vi "run.vi"(8 "error in (no error)":errorcluster, 11 "ImagingModeDL090130Frame in":refnum<class "ImagingModeDL090130Frame.lvclass">=refnum) -> (0 "error out":errorcluster, 3 "ImagingModeDL090130Frame out":refnum<class "ImagingModeDL090130Frame.lvclass">)   [LabVIEW 2010, in "ImagingModeDL090130Frame.lvclass"]
uses:
  ImagingModeDL090130Frame.lvclass
  internal_trigger_enum.ctl
  main/labview_source/controls/undock_button.ctl
  translation_mode_enum.ctl
  common/xcontrols/XSettings/XSettings/XSettings.xctl
  common/classes/GenericComponent/GenericComponent/GenericComponent.lvclass
  common/xcontrols/XIntensityCompensation/XIntensityCompensation/XIntensityCompensation.xctl
  speed_constant_enum.ctl
  control_refs.ctl
  state_enum.ctl
  common/classes/GenericToplevelComponent/GenericToplevelComponent/trigger_type_enum.ctl
  GenericImagingMode/GenericImagingMode/GenericImagingMode.lvclass
  ImagingModeDL090130Frame.lvclass/ImagingModeDL090130Frame.ctl
  Trajectory/GenericTrajectory/GenericTrajectory/GenericTrajectory.lvclass
  common/classes/ErrorController/ErrorController/class_data.vi
  common/classes/ErrorController/ErrorController/ErrorController.lvclass
panel:
  out "enforce settings?":bool
  in  "button:undock":T1
  in  "Tab Control":enum32{"User", "Debug", "About"}(tab)
  in  "amplitude\n (y galvo, V)":dbl(slide)=1.0 min=0.0 max=4.0 step=0.01 scale=0.0..4.0
  in  "center\n (y galvo, V)":dbl(slide) min=-2.0 max=2.0 step=0.01 scale=-2.0..2.0
  in  "amplitude\n (x galvo, V)":dbl(slide)=1.0 min=0.0 max=4.0 step=0.01 scale=0.0..4.0
  in  "center\n (x galvo, V)":dbl(slide)=1.1102230246251565e-16 min=-2.0 max=2.0 step=0.01 scale=-2.0..2.0
  in  "XIntensityCompensation":cluster{"A":dbl, "lambda":dbl[unit], "C":dbl}(xcontrol)
  in  "translation mode":T2
  in  "return to origin?":bool=TRUE
  in  "step":dbl[unit] min=0.0 max=0.01 step=1e-07
  in  "no. of averagings":i32=1 caption="repetitions/\naveraging" min=1 max=100000000
  in  "movie duration":dbl[unit]=10.24 min=0.0 max=3600.0
  in  "no. of frames":i32=20 caption="frames" min=1 max=100000
  in  "defineButton":bool
  in  "frame rate":dbl[unit]=1.953125 min=0.0 max=100.0
  in  "pixel dwell time":dbl[unit]=7.8125e-06 min=0.0 max=0.001
  in  "line scan time":dbl[unit]=0.002 min=0.0 max=1.0
  in  "y aspect":dbl=1.0 caption=":" min=0.0
  in  "x aspect":dbl=1.0 caption="aspect ratio (x:y)" min=0.0 step=1.0
  in  "y lines":i32=256 min=0 max=1000
  out "offset":dbl[unit]
  in  "x pixels":i32=256 min=0 max=1000 step=1
  out "frame no.":i32=12 caption="frame"
  out "repetition no.":i32=1 caption="repetition"
  in  "settings":refnum<class "GenericComponent.lvclass">(xcontrol)
  in  "keep constant":T3
  out "Vmax(ygalvo)":dbl
  out "Vmin(ygalvo)":dbl
  out "Vmax(xgalvo)":dbl
  out "Vmin(xgalvo)":dbl
  in  "xy galvo view?":bool
  out "event handling loop counter":i32=10
  out "statemachine loop counter":i32=75
  out "event error":errorcluster
  out "action handler error":errorcluster
  out "finished?":bool
  out "last trigger":T4
  out "internal triggers":T4[](array[typedef])
  # "stack settings"
  # "y galvo:"
  # "frame settings"
  # "TAG lens:"
  # "x galvo:"
  # "in fact 2x"
  # "current values"
  # "if no extra lines\nframe rate x2"
  # "ImagingModeDL090130Frame"
  # "Implemented by: \nDominik Langer, University of Zurich"
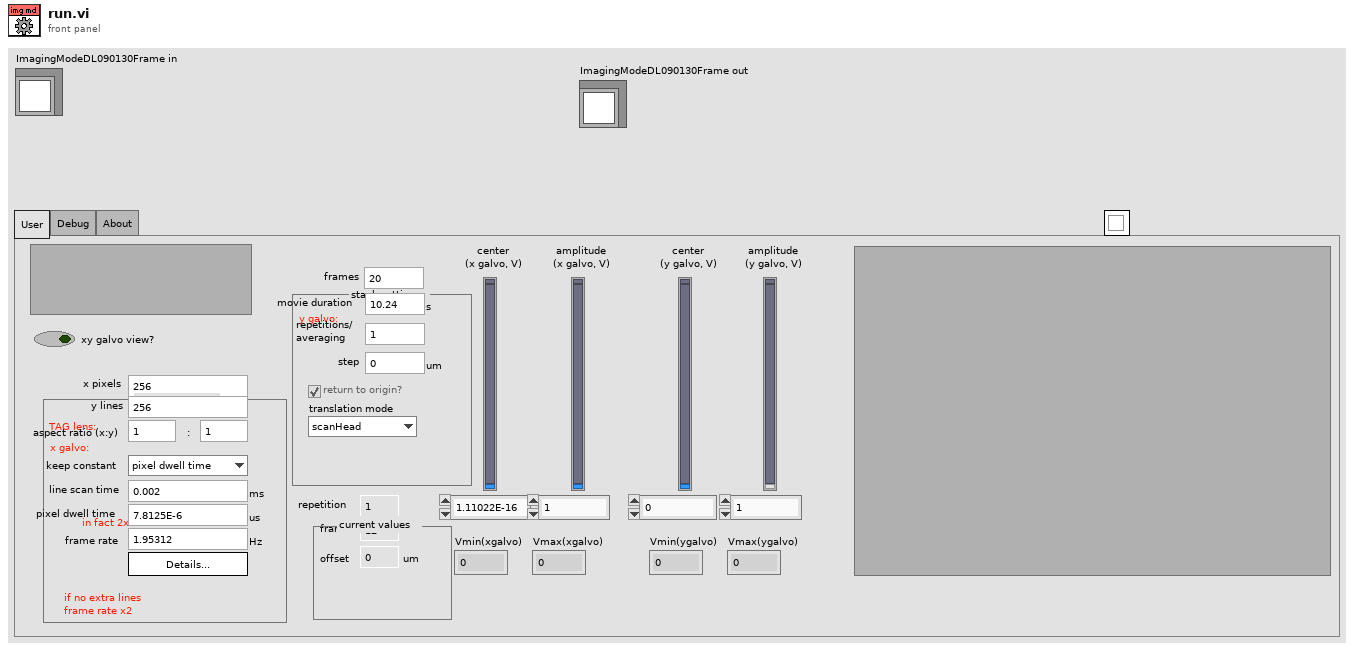
[diagram p1: front panel]
types:
  T1 = typedef "undock_button.ctl" = bool
  T2 = typedef "ImagingModeDL090130Frame.lvclass/translation_mode_enum.ctl" = enum16{"scanHead", "stage"}
  T3 = typedef "ImagingModeDL090130Frame.lvclass/speed_constant_enum.ctl" = enum16{"pixel dwell time", "line scan time", "frame rate"}
  T4 = typedef "ImagingModeDL090130Frame.lvclass/internal_trigger_enum.ctl" = enum16{"NULL", "initialise", "terminate", "start", "stop", "proceed", "update", "translate", "start scanning"}
  T5 = typedef "ImagingModeDL090130Frame.lvclass/control_refs.ctl" = cluster{"resolution controls":cluster{"x pixels":refnum<vi>, "y pixels":refnum<vi>, "ratio x factor":refnum<vi>, "ratio y factor":refnum<vi>, "center(xgalvo,V)":refnum<vi>, "center(ygalvo,V)":refnum<vi>, "amplitude(ygalvo,V)":refnum<vi>, "amplitude(xgalvo,V)":refnum<vi>, "xy galvo view?":refnum<vi>}, "speed controls":cluster{"pixel dwell time":refnum<vi>, "line scan time":refnum<vi>, "frame rate":refnum<vi>, "keep constant":refnum<vi>}, "number of frames controls":cluster{"# of frames":refnum<vi>, "duration":refnum<vi>, "# of repetitions":refnum<vi>}, "current value indicators":cluster{"frame #":refnum<vi>, "repetition #":refnum<vi>, "offset":refnum<vi>}, "step controls":cluster{"step size":refnum<vi>, "return to origin?":refnum<vi>, "translation mode":refnum<vi>, "XIntensityCompensation":refnum<vi>}, "defineButton":refnum<vi>, "settings enforced?":refnum<vi>, "settings":refnum<vi>}
  T6 = typedef "ImagingModeDL090130Frame.lvclass/state_enum.ctl" = enum16{"idle", "sweep (scanning)", "sweep (translating)"}
  T7 = typedef "trigger_type_enum.ctl" = enum8{"external", "internal", "common"}
  T8 = typedef "main_trigger_enum.ctl" = enum16{"NULL", "initialise", "terminate", "start", "stop", "change objective", "change experimentController", "change imagingMode", "save notebook", "started saving", "finished saving", "expCtr ready", "expCtr missing", "imgMd ready", "imgMd missing", "scanHd ready", "scanHd missing", "DAQ ready", "DAQ missing", "imgAsm ready", "imgAsm missing", "dataColl ready", "dataColl missing", "display ready", "display missing", "analysr ready", "analysr missing", "instrmnt ready", "instrmnt missing", "stimltr ready", "stimltr missing", "stage ready", "stage missing"}
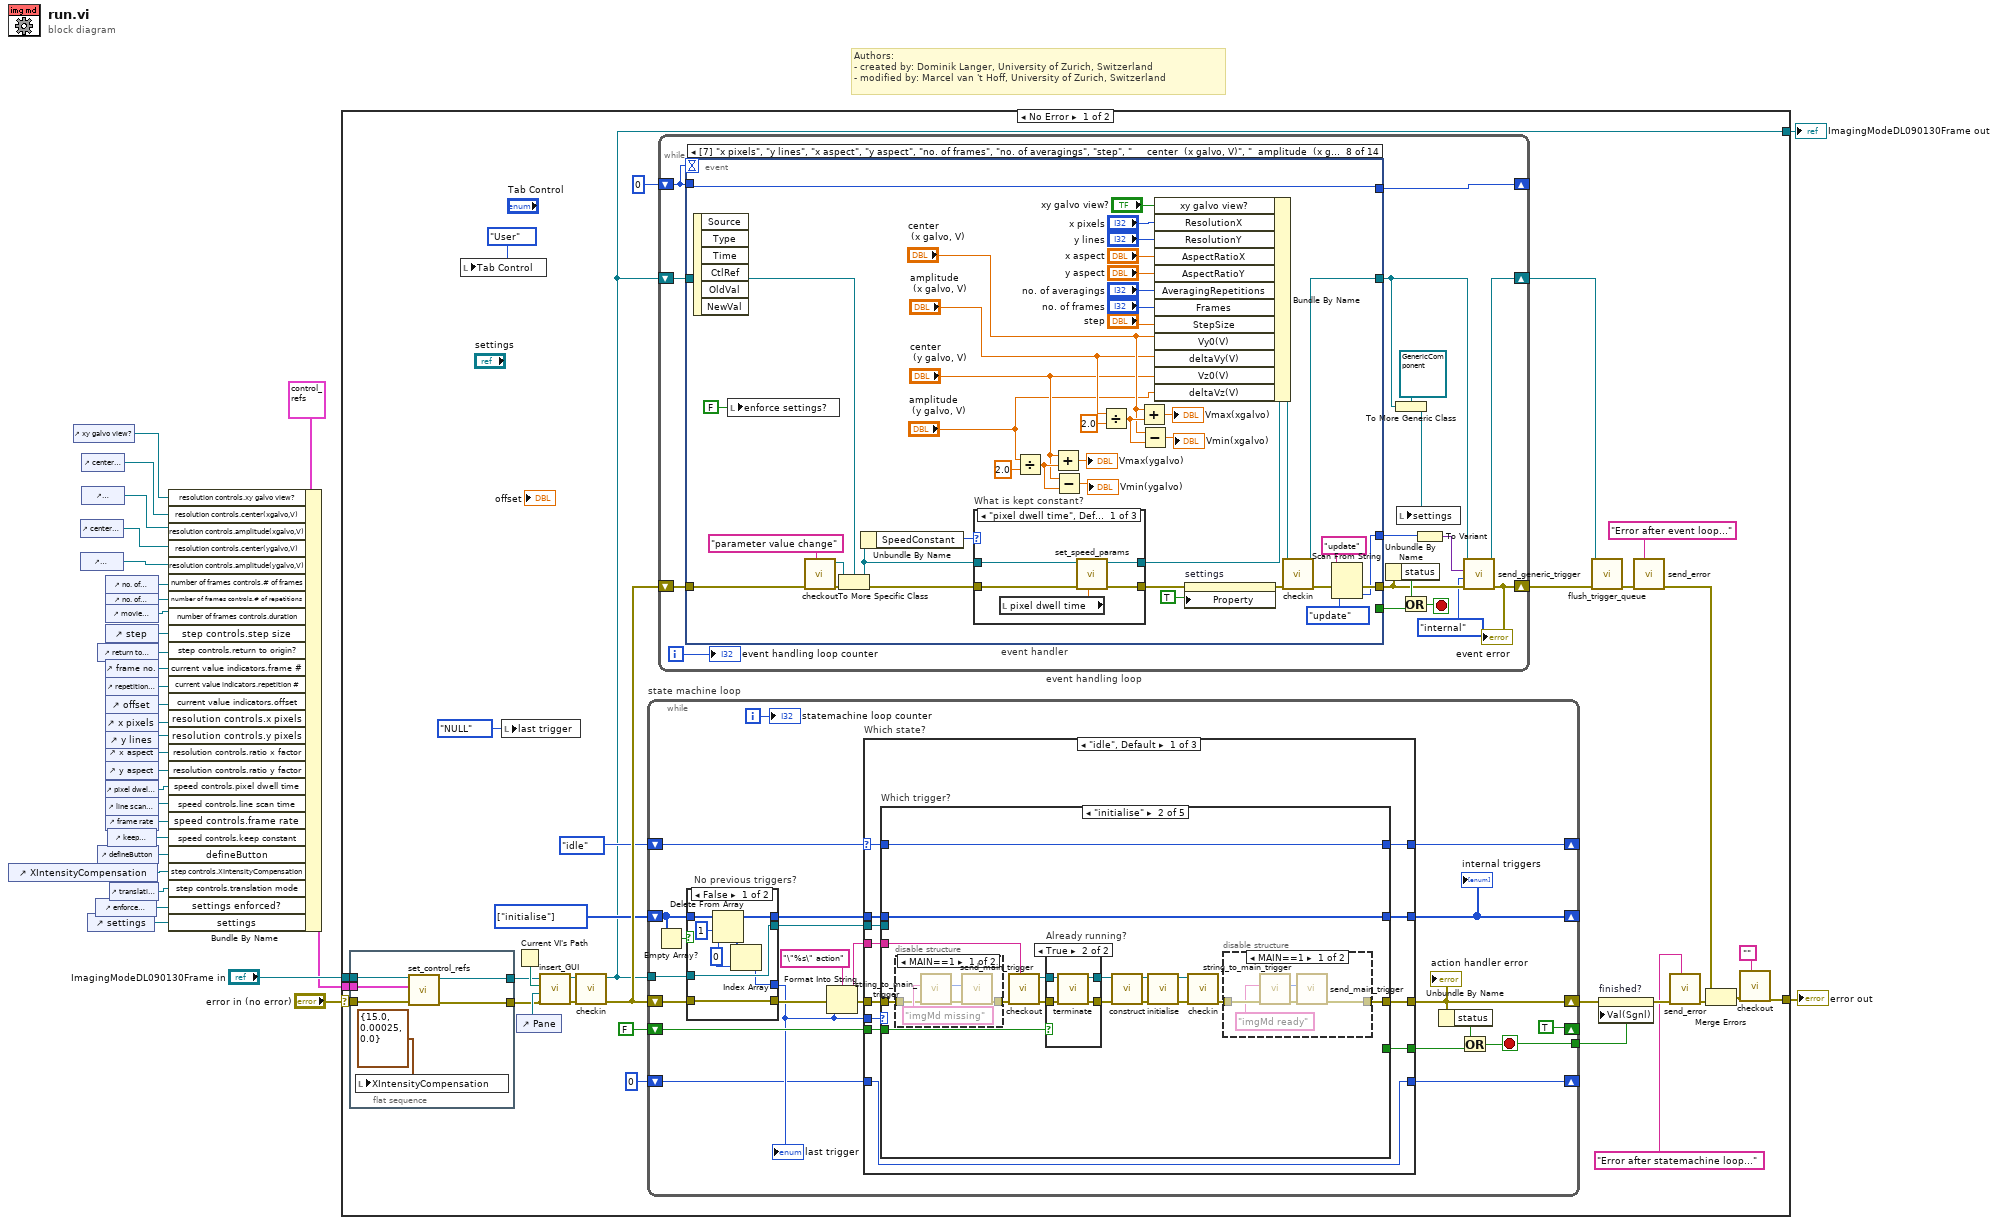
[diagram p0: block diagram]
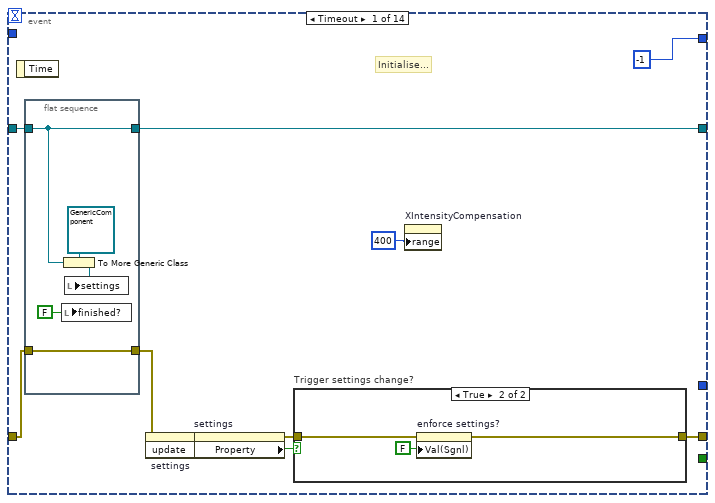
[diagram p2: hidden frame]
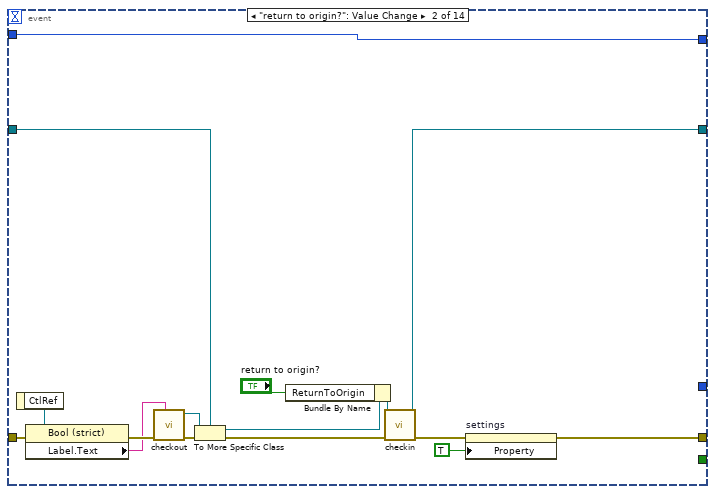
[diagram p4: hidden frame]
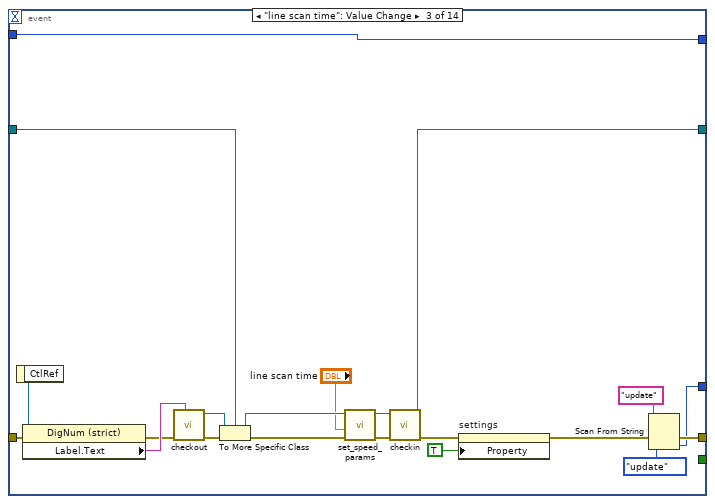
[diagram p5: hidden frame]
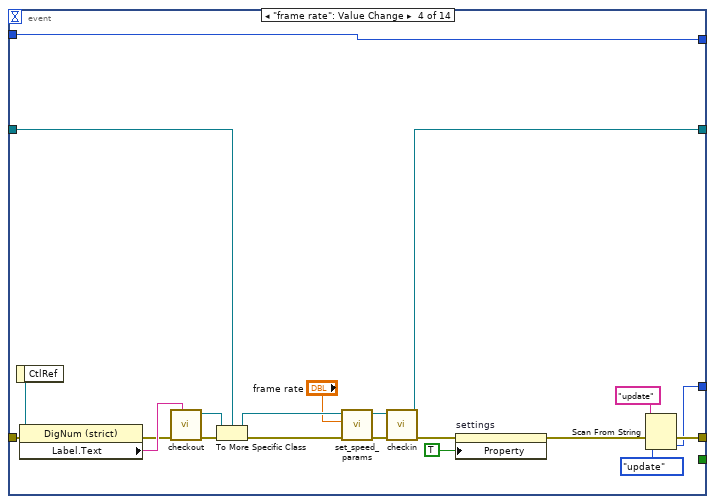
[diagram p6: hidden frame]
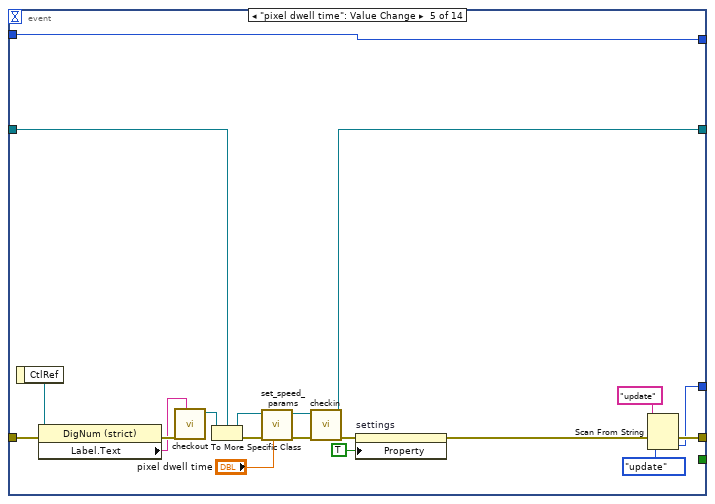
[diagram p7: hidden frame]
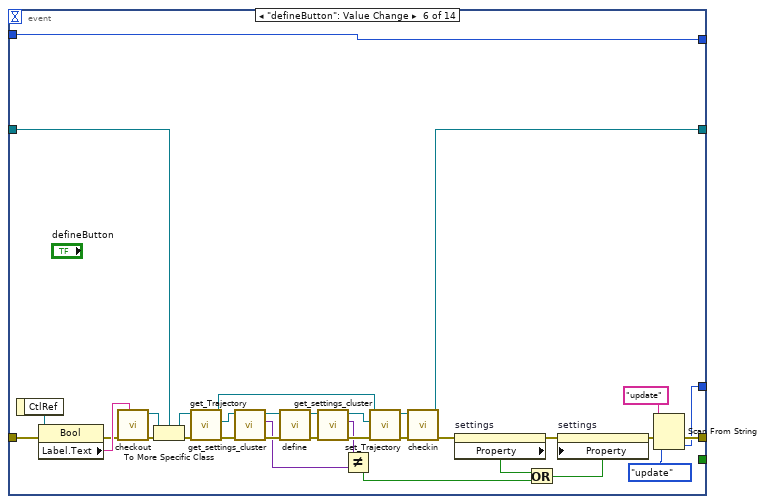
[diagram p8: hidden frame]
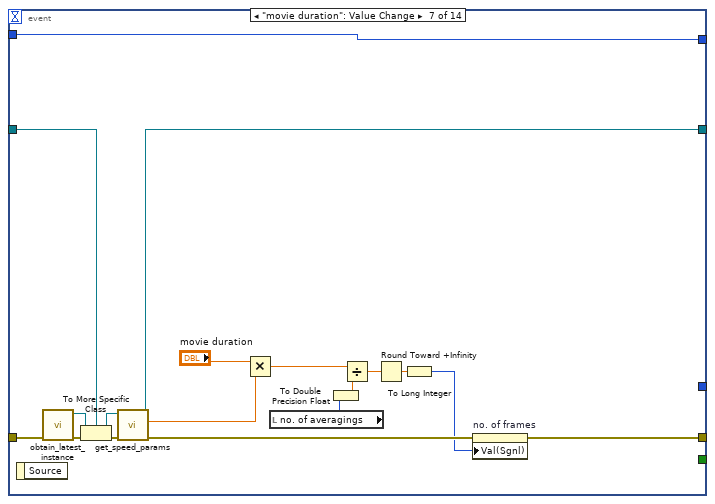
[diagram p9: hidden frame]
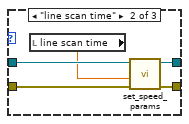
[diagram p10: hidden frame]
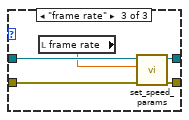
[diagram p11: hidden frame]
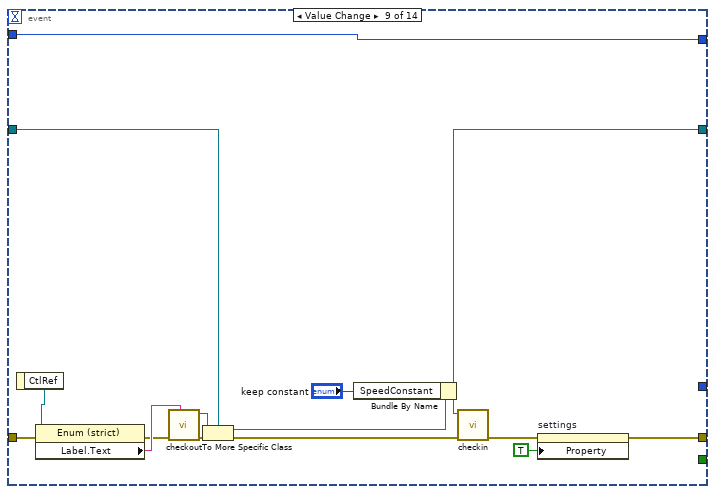
[diagram p12: hidden frame]
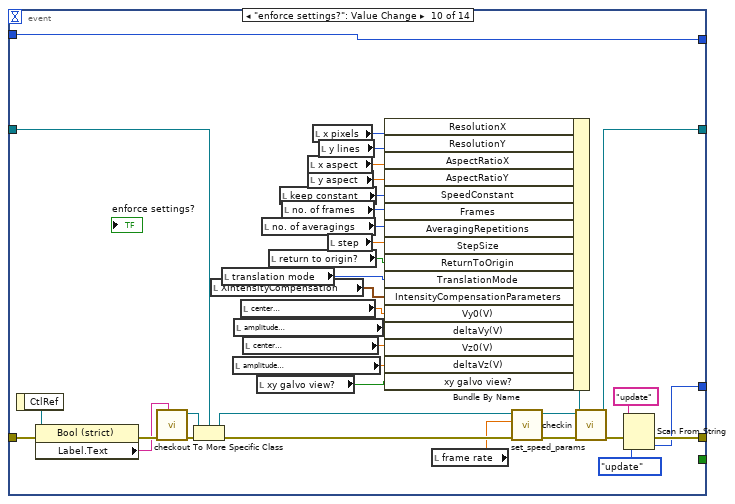
[diagram p13: hidden frame]
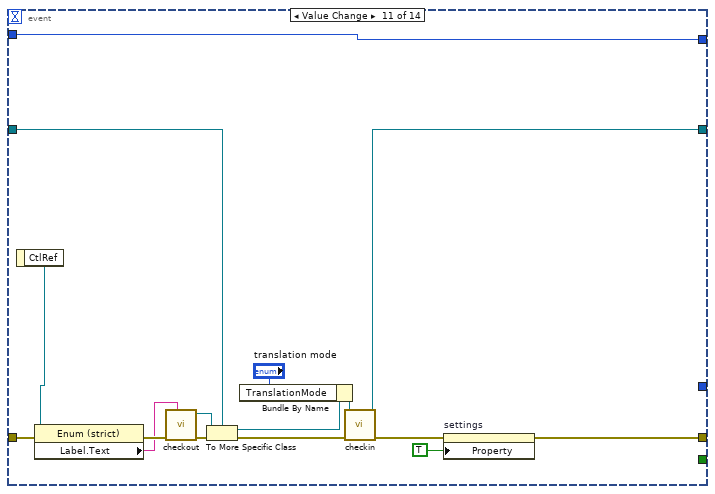
[diagram p14: hidden frame]
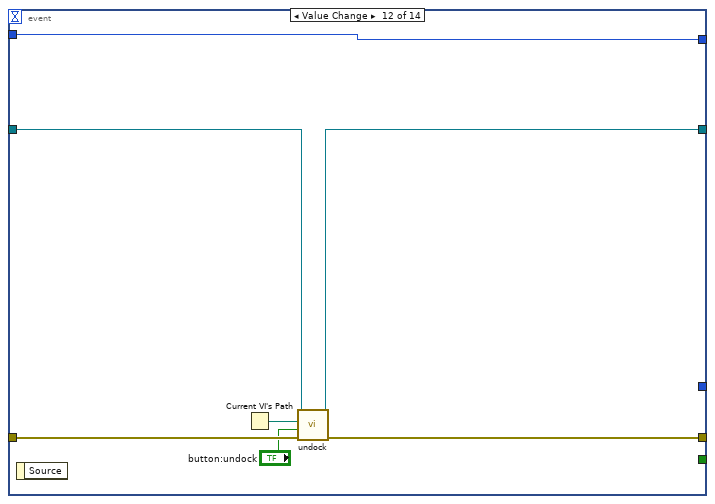
[diagram p15: hidden frame]
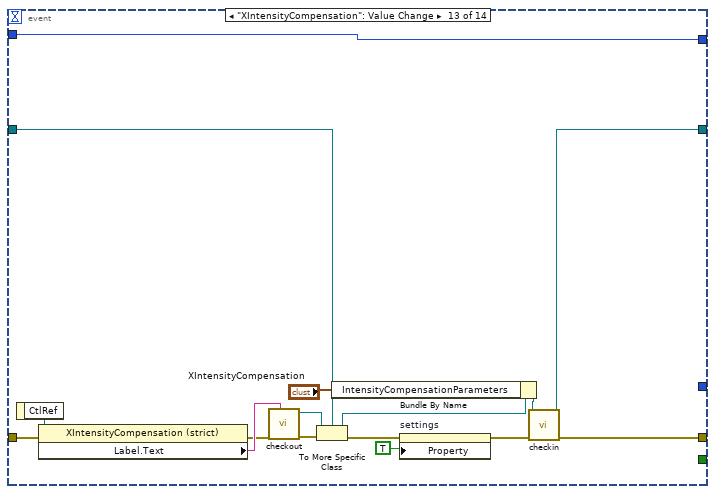
[diagram p16: hidden frame]
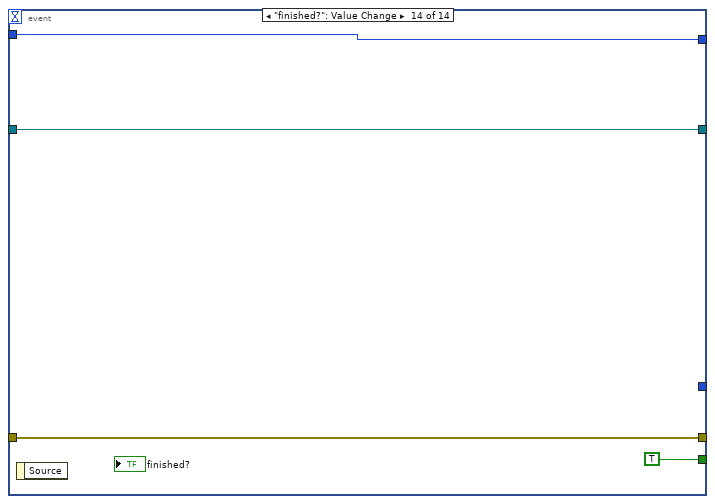
[diagram p17: hidden frame]
diagram:
  # "Authors: \n- created by: Dominik Langer, University of Zurich, Switzerland\n- modified by: Marcel van 't Hoff, University of Zurich, Switzerland"
  n1 = control-ref of="XIntensityCompensation"() -> (w10:refnum<vi>)
  n2 = control-ref of="xy galvo view?"() -> (w1:refnum<vi>)
  n3 = control-ref of="center\n (y galvo, V)"() -> (w4:refnum<vi>)
  n4 = control-ref of="amplitude\n (y galvo, V)"() -> (w3:refnum<vi>)
  n5 = control-ref of="center\n (x galvo, V)"() -> (w2:refnum<vi>)
  n6 = control-ref of="amplitude\n (x galvo, V)"() -> (w5:refnum<vi>)
  n7 = control-ref of="settings"() -> (w6:refnum<vi>)
  n8 = control-ref of="enforce settings?"() -> (w8:refnum<vi>)
  n9 = control-ref of="return to origin?"() -> (w11:refnum<vi>)
  n10 = control-ref of="defineButton"() -> (w20:refnum<vi>)
  n11 = control-ref of="no. of frames"() -> (w16:refnum<vi>)
  n12 = control-ref of="no. of averagings"() -> (w14:refnum<vi>)
  n13 = control-ref of="movie duration"() -> (w15:refnum<vi>)
  n14 = control-ref of="step"() -> (w13:refnum<vi>)
  n15 = control-ref of="frame no."() -> (w27:refnum<vi>)
  n16 = control-ref of="repetition no."() -> (w28:refnum<vi>)
  n17 = control-ref of="offset"() -> (w30:refnum<vi>)
  n18 = control-ref of="x pixels"() -> (w29:refnum<vi>)
  n19 = control-ref of="y lines"() -> (w23:refnum<vi>)
  n20 = control-ref of="x aspect"() -> (w22:refnum<vi>)
  n21 = control-ref of="y aspect"() -> (w21:refnum<vi>)
  n22 = control-ref of="pixel dwell time"() -> (w17:refnum<vi>)
  n23 = control-ref of="line scan time"() -> (w18:refnum<vi>)
  n24 = control-ref of="frame rate"() -> (w19:refnum<vi>)
  n25 = control-ref of="keep constant"() -> (w7:refnum<vi>)
  n26 = control-ref of="translation mode"() -> (w12:refnum<vi>)
  n27 = Bundle By Name(cluster=T5 {"resolution controls"={"x pixels"=refnum, "y pixels"=refnum, "ratio x factor"=refnum, "ratio y factor"=refnum, "center(xgalvo,V)"=refnum, "center(ygalvo,V)"=refnum, "amplitude(ygalvo,V)"=refnum, "amplitude(xgalvo,V)"=refnum, "xy galvo view?"=refnum}, "speed controls"={"pixel dwell time"=refnum, "line scan time"=refnum, "frame rate"=refnum, "keep constant"=refnum}, "number of frames controls"={"# of frames"=refnum, "duration"=refnum, "# of repetitions"=refnum}, "current value indicators"={"frame #"=refnum, "repetition #"=refnum, "offset"=refnum}, "step controls"={"step size"=refnum, "return to origin?"=refnum, "translation mode"=refnum, "XIntensityCompensation"=refnum}, "defineButton"=refnum, "settings enforced?"=refnum, "settings"=refnum} ("control refs"), "resolution controls.xy galvo view?"=w1, "resolution controls.center(xgalvo,V)"=w2, "resolution controls.amplitude(xgalvo,V)"=w5, "resolution controls.center(ygalvo,V)"=w4, "resolution controls.amplitude(ygalvo,V)"=w3, "number of frames controls.# of frames"=w16, "number of frames controls.# of repetitions"=w14, "number of frames controls.duration"=w15, "step controls.step size"=w13, "step controls.return to origin?"=w11, "current value indicators.frame #"=w27, "current value indicators.repetition #"=w28, "current value indicators.offset"=w30, "resolution controls.x pixels"=w29, "resolution controls.y pixels"=w23, "resolution controls.ratio x factor"=w22, "resolution controls.ratio y factor"=w21, "speed controls.pixel dwell time"=w17, "speed controls.line scan time"=w18, "speed controls.frame rate"=w19, "speed controls.keep constant"=w7, "defineButton"=w20, "step controls.XIntensityCompensation"=w10, "step controls.translation mode"=w12, "settings enforced?"=w8, "settings"=w6) -> (w24:T5)
  n28 = case shown="No Error" "error in (no error)" {
    selector: "error in (no error)" -> [w48 w659]
    tunnel: [w51 w659] -> w32
    tunnel: [w35 w658] -> w31
    tunnel: "ImagingModeDL090130Frame in" -> [w44 w658]
    tunnel: w24 -> [w45 _]
    frame No Error {
      w39 = T4[] [enum."initialise"] items=["NULL", "initialise", "terminate", "start", "stop", "proceed", "update", "translate", "start scanning"]
      n29 = flat-sequence {
        tunnel: w48 -> [w69]
        tunnel: [w68] -> w47
        tunnel: [w67] -> w46
        tunnel: w45 -> [w66]
        tunnel: w44 -> [w65]
        frame #0 {
          n30 = local write "XIntensityCompensation"(cluster{"A":dbl, "lambda":dbl[unit], "C":dbl} {"A"=15.0, "lambda"=0.00025, "C"=0.0} ("XIntensityCompensation")) -> ()
          n31 = call "set_control_refs.vi"("error in (no error)"=w69, "control refs"=w66, "ImagingModeDL090130Frame in"=w65) -> ("error out"=w67:errorcluster, "ImagingModeDL090130Frame out"=w68:refnum<class "ImagingModeDL090130Frame.lvclass">)  [unwired: 7 in]
        }
      }
      n32 = local write "Tab Control"(enum32{"User", "Debug", "About"}."User" ("Tab Control")) -> ()
      n33 = local write "last trigger"(internal_trigger_enum."NULL" ("last trigger")) -> ()
      n34 = Current VI's Path() -> (path=w59:path)
      n35 = control-ref of="Pane"() -> (w57:refnum<vi>)
      n36 = call-dynamic "insert_GUI.vi"("error in (no error)"=w46, "Pane"=w57, "VI path"=w59, "GenericComponent in"=w47) -> ("error out"=w34:errorcluster, "GenericComponent out"=w43:refnum<class "ImagingModeDL090130Frame.lvclass">)  [unwired: 6 in]
      n37 = call-dynamic "checkin.vi"("error in (no error)"=w34, "GenericScanMode in"=w43) -> ("error out"=w60:errorcluster, "GenericScanMode out"=w35:refnum<class "ImagingModeDL090130Frame.lvclass">)  [unwired: 8 in]
      n38 = while "state machine loop" {
        shift-right: [TRUE] -> _
        shift-left: FALSE -> [w396]
        tunnel: w35 -> [w407]
        tunnel: [w405] -> w42
        shift-right: [w402] -> w61
        shift-left: w60 -> [w406]
        shift-right: [w392] -> _
        shift-left: w39 -> [w394]
        shift-right: [w390] -> _
        shift-left: state_enum."idle" ("state") -> [w391]
        shift-right: [w386] -> _
        shift-left: u32 0 ("millisecond timer value") -> [w387]
        i -> [w388]
        stop <- w405 stop-if-true
        n39 = Empty Array?(array=w394) -> (empty?=w395:bool)
        n40 = case "No previous triggers?" shown="False" w395 {
          tunnel: w407 -> [w649 w657]
          tunnel: w406 -> [w651 w656]
          tunnel: [w649 w655] -> w404
          tunnel: [w644 w654] -> w389
          tunnel: [w651 w653] -> w400
          tunnel: w394 -> [w650 w652]
          tunnel: [w647 w652] -> w393
          frame False {
            w645 = 0 ("index")
            n41 = Delete From Array(array=w650, length=1, index=w645) -> (deleted portion=w646:T4[], array with subset deleted=w647:T4[])
            n42 = Index Array(array=w646, index=w645) -> (element=w644:T4)
          }
          frame True {
            n43 = call-dynamic "fetch_and_translate_trigger.vi"("error in (no error)"=w656, "ImagingModeDL090130Frame in"=w657) -> ("error out"=w653:errorcluster, "internal trigger"=w654:T4, "ImagingModeDL090130Frame out"=w655:refnum<class "ImagingModeDL090130Frame.lvclass">)  [unwired: 6 in, 1 out]
          }
        }
        "last trigger" <- w389
        n44 = Format Into String(format string="\"%s\" action", error in=w400, w389) -> (resulting string=w398:string, error out=w399:errorcluster)  [unwired: 1 in]
        n45 = case "Which state?" shown="\"idle\", Default" w391 {
          selector: w391 -> [w411 w505 w616]
          tunnel: w404 -> [w420 w508 w609]
          tunnel: [w419 _ _] -> w403
          tunnel: [w418 w510 w611] -> w402
          tunnel: w399 -> [w417 w511 w613]
          tunnel: w398 -> [w416 w507 w608]
          tunnel: w396 -> [w415 _ _]
          tunnel: w393 -> [w414 w509 w614]
          tunnel: w389 -> [w413 w503 w612]
          tunnel: [w412 w506 w610] -> w392
          tunnel: [w410 w504 w615] -> w390
          tunnel: w387 -> [w409 w502 w607]
          tunnel: [w409 w501 w607] -> w386
          frame "idle", Default {
            n46 = case "Which trigger?" shown="\"initialise\"" w413 {
              tunnel: w417 -> [w423 w425 w461 w482 w492]
              tunnel: w420 -> [_ _ _ w479 w490]
              tunnel: [w423 w427 w459 w481 w491] -> w418
              tunnel: [_ _ TRUE _ _] -> w419
              tunnel: w414 -> [w422 w439 w467 w478 w500]
              tunnel: [w422 w439 w467 w477 w500] -> w412
              tunnel: w416 -> [_ w436 w462 w480 w493]
              tunnel: w415 -> [_ w429 _ _ _]
              tunnel: [w421 w426 w458 state_enum."sweep (scanning)" ("state") w489] -> w410
              tunnel: w411 -> [w421 w426 w458 _ w489]
              frame "NULL", Default {
              }
              frame "initialise" {
                n47 = disable-structure shown="MAIN==1" {
                  disable-tunnel: w425 -> [w440 w445]
                  disable-tunnel: [w444 w445] -> w424
                  frame condition #0 {
                    n48 = call "string_to_main_trigger.vi"("error in (no error)"=w440, "trigger string"="imgMd missing") -> ("error out"=w443:errorcluster, "main trigger"=w442:T8)  [unwired: 8 in]
                    n49 = call "send_main_trigger.vi"("error in (no error)"=w443, "trigger"=w442) -> ("error out"=w444:errorcluster)  [unwired: 9 in]
                  }
                  frame condition #1 (active) {
                  }
                }
                n50 = call "checkout.vi"("locked by?"=w436, "error in (no error)"=w424) -> ("error out"=w433:errorcluster, "GenericScanMode out"=w432:refnum<class "GenericImagingMode.lvclass">)  [unwired: 8 in]
                n51 = case "Already running?" shown="True" w429 {
                  tunnel: w433 -> [w453 w457]
                  tunnel: w432 -> [w452 w456]
                  tunnel: [w452 w455] -> w431
                  tunnel: [w453 w454] -> w430
                  frame False {
                  }
                  frame True {
                    n52 = call-dynamic "terminate.vi"("error in (no error)"=w457, "GenericPlugin in"=w456) -> ("error out"=w454:errorcluster, "GenericPlugin out"=w455:refnum<class "GenericImagingMode.lvclass">)  [unwired: 8 out]
                  }
                }
                n53 = call-dynamic "construct.vi"("error in (no error)"=w430, "GenericPlugin in"=w431) -> ("error out"=w435:errorcluster, "GenericPlugin out"=w438:refnum<class "GenericImagingMode.lvclass">)  [unwired: 2 in, 6 out]
                n54 = call-dynamic "initialise.vi"("error in (no error)"=w435, "GenericPlugin in"=w438) -> ("error out"=w434:errorcluster, "GenericPlugin out"=w437:refnum<class "GenericImagingMode.lvclass">)  [unwired: 8 out]
                n55 = call-dynamic "checkin.vi"("error in (no error)"=w434, "GenericScanMode in"=w437) -> ("error out"=w428:errorcluster)  [unwired: 8 in, 1 out]
                n56 = disable-structure shown="MAIN==1" {
                  disable-tunnel: w428 -> [w449 w451]
                  disable-tunnel: [w450 w451] -> w427
                  frame condition #0 {
                    n57 = call "string_to_main_trigger.vi"("error in (no error)"=w449, "trigger string"="imgMd ready") -> ("error out"=w448:errorcluster, "main trigger"=w447:T8)  [unwired: 8 in]
                    n58 = call "send_main_trigger.vi"("error in (no error)"=w448, "trigger"=w447) -> ("error out"=w450:errorcluster)  [unwired: 9 in]
                  }
                  frame condition #1 (active) {
                  }
                }
              }
              frame "terminate" {
                n59 = disable-structure shown="MAIN==1" {
                  disable-tunnel: w461 -> [w472 w474]
                  disable-tunnel: [w473 w474] -> w460
                  frame condition #0 {
                    n60 = call "string_to_main_trigger.vi"("error in (no error)"=w472, "trigger string"="imgMd missing") -> ("error out"=w470:errorcluster, "main trigger"=w471:T8)  [unwired: 8 in]
                    n61 = call "send_main_trigger.vi"("error in (no error)"=w470, "trigger"=w471) -> ("error out"=w473:errorcluster)  [unwired: 9 in]
                  }
                  frame condition #1 (active) {
                  }
                }
                n62 = call "checkout.vi"("locked by?"=w462, "error in (no error)"=w460) -> ("error out"=w464:errorcluster, "GenericScanMode out"=w466:refnum<class "GenericImagingMode.lvclass">)  [unwired: 8 in]
                n63 = call-dynamic "terminate.vi"("error in (no error)"=w464, "GenericPlugin in"=w466) -> ("error out"=w463:errorcluster, "GenericPlugin out"=w465:refnum<class "GenericImagingMode.lvclass">)  [unwired: 8 out]
                n64 = call-dynamic "checkin.vi"("error in (no error)"=w463, "GenericScanMode in"=w465) -> ("error out"=w459:errorcluster)  [unwired: 8 in, 1 out]
              }
              frame "start" {
                n65 = call "checkout.vi"("locked by?"=w480, "error in (no error)"=w482) -> ("error out"=w483:errorcluster, "GenericScanMode out"=w484:refnum<class "GenericImagingMode.lvclass">)  [unwired: 8 in]
                n66 = To More Specific Class(target class=w479, reference=w484, error in=w483) -> (specific class reference=w487:refnum<class "ImagingModeDL090130Frame.lvclass">, error out=w488:errorcluster)
                n67 = call-dynamic "start_sweep.vi"("error in (no error)"=w488, "ImagingModeDL090130Frame in"=w487) -> ("error out"=w486:errorcluster, "ImagingModeDL090130Frame out"=w485:refnum<class "ImagingModeDL090130Frame.lvclass">)  [unwired: 8 out]
                n68 = call-dynamic "checkin.vi"("error in (no error)"=w486, "GenericScanMode in"=w485) -> ("error out"=w481:errorcluster)  [unwired: 8 in, 1 out]
                n69 = Build Array (concatenate)(w478, internal_trigger_enum."start scanning" ("internal trigger")) -> (w477:T4[])
              }
              frame "update" {
                n70 = call "checkout.vi"("locked by?"=w493, "error in (no error)"=w492) -> ("error out"=w494:errorcluster, "GenericScanMode out"=w495:refnum<class "GenericImagingMode.lvclass">)  [unwired: 8 in]
                n71 = To More Specific Class(target class=w490, reference=w495, error in=w494) -> (specific class reference=w499:refnum<class "ImagingModeDL090130Frame.lvclass">, error out=w496:errorcluster)
                n72 = call-dynamic "update.vi"("error in (no error)"=w496, "ImagingModeDL090130Frame in"=w499) -> ("error out"=w497:errorcluster, "ImagingModeDL090130Frame out"=w498:refnum<class "ImagingModeDL090130Frame.lvclass">)  [unwired: 8 out]
                n73 = call-dynamic "checkin.vi"("error in (no error)"=w497, "GenericScanMode in"=w498) -> ("error out"=w491:errorcluster)  [unwired: 8 in, 1 out]
              }
            }
          }
          frame "sweep (scanning)" {
            n74 = case "Which action?" shown="\"NULL\", Default" w503 {
              tunnel: w511 -> [w515 w529 w539 w597]
              tunnel: w508 -> [_ w530 w540 w599]
              tunnel: [w515 w528 w538 w596] -> w510
              tunnel: w509 -> [w514 w526 w536 w606]
              tunnel: [w514 w526 w535 w606] -> w506
              tunnel: w507 -> [_ w527 w537 w598]
              tunnel: w505 -> [w513 _ w534 w595]
              tunnel: [w513 state_enum."idle" ("state") w533 w595] -> w504
              tunnel: w502 -> [w512 w516 w532 w594]
              tunnel: [w512 w516 w531 w594] -> w501
              frame "NULL", Default {
              }
              frame "stop" {
                n75 = call "checkout.vi"("locked by?"=w527, "error in (no error)"=w529) -> ("error out"=w523:errorcluster, "GenericScanMode out"=w524:refnum<class "GenericImagingMode.lvclass">)  [unwired: 8 in]
                n76 = To More Specific Class(target class=w530, reference=w524, error in=w523) -> (specific class reference=w521:refnum<class "ImagingModeDL090130Frame.lvclass">, error out=w519:errorcluster)
                n77 = call-dynamic "stop_scanning.vi"("error in (no error)"=w519, "ScanModeDL090923Scaffold in"=w521) -> ("error out"=w518:errorcluster, "ScanModeDL090923Scaffold out"=w520:refnum<class "ImagingModeDL090130Frame.lvclass">)  [unwired: 8 out]
                n78 = call-dynamic "stop_sweep.vi"("error in (no error)"=w518, "ImagingModeDL090130Frame in"=w520) -> ("error out"=w522:errorcluster, "ImagingModeDL090130Frame out"=w525:refnum<class "ImagingModeDL090130Frame.lvclass">)  [unwired: 8 in]
                n79 = call-dynamic "checkin.vi"("error in (no error)"=w522, "GenericScanMode in"=w525) -> ("error out"=w528:errorcluster)  [unwired: 8 in, 1 out]
              }
              frame "proceed" {
                n80 = call "checkout.vi"("locked by?"=w537, "error in (no error)"=w539) -> ("error out"=w541:errorcluster, "GenericScanMode out"=w542:refnum<class "GenericImagingMode.lvclass">)  [unwired: 8 in]
                n81 = To More Specific Class(target class=w540, reference=w542, error in=w541) -> (specific class reference=w543:refnum<class "ImagingModeDL090130Frame.lvclass">, error out=w544:errorcluster)
                n82 = call-dynamic "get_number_of_frames.vi"("error in (no error)"=w544, "ImagingModeDL090130Frame in"=w543) -> ("error out"=w546:errorcluster, "number of frames"=w545:i32, "ImagingModeDL090130Frame out"=w547:refnum<class "ImagingModeDL090130Frame.lvclass">)  [unwired: 7 out]
                n83 = case "Focus or stack/movie mode?" shown="Default" w545 {
                  tunnel: [w554 w567] -> w548
                  tunnel: w536 -> [w553 w573]
                  tunnel: [w553 w572] -> w535
                  tunnel: w546 -> [w554 w569]
                  tunnel: w547 -> [w552 w568]
                  tunnel: [w552 w561] -> w549
                  tunnel: w534 -> [w551 w566]
                  tunnel: [w551 w565] -> w533
                  tunnel: w532 -> [w550 w558]
                  tunnel: [w550 w560] -> w531
                  frame -1 {
                    # "Focus mode: don't react..."
                  }
                  frame Default {
                    # "Stack/movie mode..."
                    n84 = call-dynamic "is_finished.vi"("error in (no error)"=w569, "ImagingModeDL090130Frame in"=w568) -> ("error out"=w571:errorcluster, "finished?"=w564:bool[], "ImagingModeDL090130Frame out"=w570:refnum<class "ImagingModeDL090130Frame.lvclass">)  [unwired: 7 out]
                    n85 = Tick Count (ms)() -> (millisecond timer value=w559:u32)
                    n86 = Subtract(x=w559, y=w558) -> (x-y=w556:u32)
                    n87 = call-dynamic "iterate.vi"("error in (no error)"=w571, "ImagingModeDL090130Frame in"=w570) -> ("error out"=w567:errorcluster, "ImagingModeDL090130Frame out"=w561:refnum<class "ImagingModeDL090130Frame.lvclass">)  [unwired: 8 out]
                    n88 = Index Array(array=w564) -> (element #1=w563:bool, element #3=w562:bool)  [unwired: 3 in, 1 out]
                    n89 = Greater?(x=w556, y=u32 100) -> (0:w557:bool)
                    n90 = case "Update indicators?" shown="False" w557 {
                      tunnel: w561 -> [_ w578]
                      tunnel: [w574 w575] -> w560
                      tunnel: w558 -> [w574 _]
                      tunnel: w559 -> [_ w575]
                      frame False {
                      }
                      frame True {
                        # "Strangely, if they are updated to often, it, it gets slowed down..."
                        n91 = Unbundle By Name(w578) -> ("current frame"=→"frame no.":i32, "current repetition"=→"repetition no.":i32)
                      }
                    }
                    n92 = case "Sweep finished?" shown="False" w563 {
                      tunnel: w573 -> [w583 w592]
                      tunnel: w562 -> [w579 _]
                      tunnel: [w582 w591] -> w572
                      tunnel: w566 -> [w581 w590]
                      tunnel: [w580 w590] -> w565
                      frame False {
                        n93 = case "scanning finished?" shown="True" w579 {
                          tunnel: w583 -> [w585 w589]
                          tunnel: [w585 w588] -> w582
                          tunnel: w581 -> [w584 _]
                          tunnel: [w584 state_enum."sweep (translating)" ("state")] -> w580
                          frame False {
                          }
                          frame True {
                            n94 = Build Array (concatenate)(w589, internal_trigger_enum."translate" ("internal trigger")) -> (w588:T4[])
                          }
                        }
                      }
                      frame True {
                        n95 = Build Array (concatenate)(w592, internal_trigger_enum."stop" ("internal trigger")) -> (w591:T4[])
                      }
                    }
                  }
                }
                n96 = call-dynamic "checkin.vi"("error in (no error)"=w548, "GenericScanMode in"=w549) -> ("error out"=w538:errorcluster)  [unwired: 8 in, 1 out]
              }
              frame "start scanning" {
                n97 = call "checkout.vi"("locked by?"=w598, "error in (no error)"=w597) -> ("error out"=w600:errorcluster, "GenericScanMode out"=w601:refnum<class "GenericImagingMode.lvclass">)  [unwired: 8 in]
                n98 = To More Specific Class(target class=w599, reference=w601, error in=w600) -> (specific class reference=w603:refnum<class "ImagingModeDL090130Frame.lvclass">, error out=w602:errorcluster)
                n99 = call-dynamic "start_scanning.vi"("error in (no error)"=w602, "ScanModeDL090923Scaffold in"=w603) -> ("error out"=w604:errorcluster, "ScanModeDL090923Scaffold out"=w605:refnum<class "ImagingModeDL090130Frame.lvclass">)  [unwired: 8 out]
                n100 = call-dynamic "checkin.vi"("error in (no error)"=w604, "GenericScanMode in"=w605) -> ("error out"=w596:errorcluster)  [unwired: 8 in, 1 out]
              }
            }
          }
          frame "sweep (translating)" {
            n101 = case "Which action?" shown="\"NULL\", Default" w612 {
              tunnel: w613 -> [w617 w624 w629 w637]
              tunnel: w609 -> [_ _ _ w636]
              tunnel: [w617 w624 w629 w635] -> w611
              tunnel: w614 -> [w619 w621 w627 w643]
              tunnel: [w619 w622 w626 w643] -> w610
              tunnel: w608 -> [_ _ _ w638]
              tunnel: w616 -> [w618 _ _ w634]
              tunnel: [w618 state_enum."sweep (scanning)" ("state") state_enum."sweep (scanning)" ("state") w634] -> w615
              frame "NULL", Default {
              }
              frame "stop" {
                n102 = Build Array (concatenate)(internal_trigger_enum."stop" ("internal trigger"), w621) -> (w622:T4[])
              }
              frame "proceed" {
                n103 = Build Array (concatenate)(w627, internal_trigger_enum."start scanning" ("internal trigger")) -> (w626:T4[])
              }
              frame "translate" {
                n104 = call "checkout.vi"("locked by?"=w638, "error in (no error)"=w637) -> ("error out"=w639:errorcluster, "GenericScanMode out"=w640:refnum<class "GenericImagingMode.lvclass">)  [unwired: 8 in]
                n105 = To More Specific Class(target class=w636, reference=w640, error in=w639) -> (specific class reference=w633:refnum<class "ImagingModeDL090130Frame.lvclass">, error out=w632:errorcluster)
                n106 = call-dynamic "stop_scanning.vi"("error in (no error)"=w632, "ScanModeDL090923Scaffold in"=w633) -> ("error out"=w631:errorcluster, "ScanModeDL090923Scaffold out"=w630:refnum<class "ImagingModeDL090130Frame.lvclass">)  [unwired: 8 out]
                n107 = call-dynamic "translate.vi"("error in (no error)"=w631, "ImagingModeDL090130Frame in"=w630) -> ("error out"=w641:errorcluster, "ImagingModeDL090130Frame out"=w642:refnum<class "ImagingModeDL090130Frame.lvclass">)  [unwired: 8 out]
                n108 = call-dynamic "checkin.vi"("error in (no error)"=w641, "GenericScanMode in"=w642) -> ("error out"=w635:errorcluster)  [unwired: 8 in, 1 out]
              }
            }
          }
        }
        "action handler error" <- w402
        "internal triggers" <- w392
        n109 = Unbundle By Name(w402) -> ("status"=w401:bool)
        n110 = Or(x=w401, y=w403) -> (x .or. y?=w405:bool)
        "statemachine loop counter" <- w388
      }
      n111 = while "event handling loop" {
        shift-right: [w85] -> _
        shift-left: 0 -> [w86]
        shift-right: [w78] -> w41
        shift-left: w60 -> [w84]
        shift-right: [w71] -> w36
        shift-left: w35 -> [w72]
        i -> [w83]
        stop <- w80 stop-if-true
        n112 = event "event handler" shown="[7] \"x pixels\", \"y lines\", \"x aspect\", \"y aspect\", \"no. of frames\", \"no. of averagings\", \"step\", \"     center\n (x galvo, V)\", \"  amplitude\n (x galvo, V) \", \"     center\n (y galvo, V)\", \"  amplitude\n (y galvo, V)\", \"xy galvo view?\": Value Change" {
          selector: _ -> [_ _ _ _ _ _ _ _ _ _ _ _ _ _]
          dyn-events: _ -> [_ _ _ _ _ _ _ _ _ _ _ _ _ _]
          timeout: w86 -> [_ _ _ _ _ _ _ _ _ _ _ _ _ _]
          tunnel: [-1 w121 w142 w163 w183 w217 w235 w276 w306 w342 w358 w365 w381 w385] -> w85
          tunnel: w86 -> [_ w121 w142 w163 w183 w217 w235 w276 w306 w342 w358 w365 w381 w385]
          tunnel: w84 -> [w95 w113 w133 w151 w175 w209 w234 w257 w296 w317 w349 w364 w372 w384]
          tunnel: [w88 w107 w127 w150 w169 w201 w219 w266 w292 w325 w343 w363 w377 w384] -> w79
          tunnel: [_ _ _ _ _ _ _ _ _ _ _ _ _ TRUE] -> w81
          tunnel: [_ _ w126 w147 w168 w200 _ w265 _ w324 _ _ _ _] -> w75
          tunnel: [w93 w111 w131 w143 w177 w205 w227 w271 w297 w314 w348 w359 w374 w382] -> w70
          tunnel: w72 -> [w94 w110 w130 w146 w172 w204 w226 w270 w301 w339 w347 w360 w373 w382]
          event Timeout {
            # "Initialise..."
            n113 = event-data() -> ()  [unwired: 2 out]
            n114 = flat-sequence {
              tunnel: w95 -> [w101]
              tunnel: w94 -> [w102]
              tunnel: [w102] -> w93
              tunnel: [w101] -> w92
              frame #0 {
                n115 = local write "finished?"(FALSE ("finished?")) -> ()
                n116 = To More Generic Class(target class=refnum<class "GenericComponent.lvclass"> refnum ("GenericComponent.lvclass"), reference=w102) -> (generic class reference=w104:refnum<class "GenericComponent.lvclass">)
                n117 = local write "settings"(w104) -> ()
              }
            }
            n118 = invoke on="settings" class="XSettings (strict)" method="update"(error in=w92) -> (error out=w91:errorcluster)  [unwired: 2 in, 2 out]
            n119 = property on="settings" class="XSettings (strict)"(error in=w91) -> (error out=w89:errorcluster, "Property"=w90:bool)  [unwired: 1 in, 1 out]
            n120 = case "Trigger settings change?" shown="True" w90 {
              tunnel: w89 -> [w97 w100]
              tunnel: [w97 w98] -> w88
              frame False {
              }
              frame True {
                n121 = property on="enforce settings?" class="Bool (strict)"(error in=w100, "Val(Sgnl)"=FALSE ("Value (Signaling)")) -> (error out=w98:errorcluster)  [unwired: 1 in, 1 out]
              }
            }
            n122 = property on="XIntensityCompensation" class="XIntensityCompensation (strict)"("range"=400) -> ()  [unwired: 2 in, 2 out]
          }
          event "return to origin?": Value Change {
            n123 = event-data() -> ("CtlRef"=w115:refnum<vi>)  [unwired: 1 out]
            n124 = property class="Bool (strict)"(reference=w115, error in=w113) -> (error out=w114:errorcluster, "Label.Text"=w112:string)  [unwired: 1 out]
            n125 = call "checkout.vi"("locked by?"=w112, "error in (no error)"=w114) -> ("error out"=w120:errorcluster, "GenericScanMode out"=w119:refnum<class "GenericImagingMode.lvclass">)  [unwired: 8 in]
            n126 = To More Specific Class(target class=w110, reference=w119, error in=w120) -> (specific class reference=w117:refnum<class "ImagingModeDL090130Frame.lvclass">, error out=w118:errorcluster)
            n127 = Bundle By Name(cluster=w117, "ReturnToOrigin"="return to origin?") -> (w116:refnum<class "ImagingModeDL090130Frame.lvclass">)
            n128 = call-dynamic "checkin.vi"("error in (no error)"=w118, "GenericScanMode in"=w116) -> ("error out"=w108:errorcluster, "GenericScanMode out"=w111:refnum<class "ImagingModeDL090130Frame.lvclass">)  [unwired: 8 in]
            n129 = property on="settings" class="XSettings (strict)"(error in=w108, "Property"=TRUE ("is user-defined?")) -> (error out=w107:errorcluster)  [unwired: 1 in, 1 out]
          }
          event "line scan time": Value Change {
            n130 = event-data() -> ("CtlRef"=w134:refnum<vi>)  [unwired: 1 out]
            n131 = property class="DigNum (strict)"(reference=w134, error in=w133) -> (error out=w132:errorcluster, "Label.Text"=w135:string)  [unwired: 1 out]
            n132 = call "checkout.vi"("locked by?"=w135, "error in (no error)"=w132) -> ("error out"=w137:errorcluster, "GenericScanMode out"=w136:refnum<class "GenericImagingMode.lvclass">)  [unwired: 8 in]
            n133 = To More Specific Class(target class=w130, reference=w136, error in=w137) -> (specific class reference=w140:refnum<class "ImagingModeDL090130Frame.lvclass">, error out=w141:errorcluster)
            n134 = call-dynamic "set_speed_params.vi"("error in (no error)"=w141, "line-scan time"="line scan time", "ImagingModeDL090130Frame in"=w140) -> ("error out"=w138:errorcluster, "ImagingModeDL090130Frame out"=w139:refnum<class "ImagingModeDL090130Frame.lvclass">)  [unwired: 7 in]
            n135 = call-dynamic "checkin.vi"("error in (no error)"=w138, "GenericScanMode in"=w139) -> ("error out"=w123:errorcluster, "GenericScanMode out"=w131:refnum<class "ImagingModeDL090130Frame.lvclass">)  [unwired: 8 in]
            n136 = property on="settings" class="XSettings (strict)"(error in=w123, "Property"=TRUE ("is user-defined?")) -> (error out=w122:errorcluster)  [unwired: 1 in, 1 out]
            n137 = Scan From String(input string="update", error in=w122, default 1=internal_trigger_enum."update" ("internal trigger")) -> (error out=w127:errorcluster, output 1=w126:T4)  [unwired: 2 in, 2 out]
          }
          event "frame rate": Value Change {
            n138 = event-data() -> ("CtlRef"=w145:refnum<vi>)  [unwired: 1 out]
            n139 = property class="DigNum (strict)"(reference=w145, error in=w151) -> (error out=w155:errorcluster, "Label.Text"=w156:string)  [unwired: 1 out]
            n140 = call "checkout.vi"("locked by?"=w156, "error in (no error)"=w155) -> ("error out"=w158:errorcluster, "GenericScanMode out"=w157:refnum<class "GenericImagingMode.lvclass">)  [unwired: 8 in]
            n141 = To More Specific Class(target class=w146, reference=w157, error in=w158) -> (specific class reference=w161:refnum<class "ImagingModeDL090130Frame.lvclass">, error out=w162:errorcluster)
            n142 = call-dynamic "set_speed_params.vi"("error in (no error)"=w162, "frame rate"="frame rate", "ImagingModeDL090130Frame in"=w161) -> ("error out"=w159:errorcluster, "ImagingModeDL090130Frame out"=w160:refnum<class "ImagingModeDL090130Frame.lvclass">)  [unwired: 7 in]
            n143 = call-dynamic "checkin.vi"("error in (no error)"=w159, "GenericScanMode in"=w160) -> ("error out"=w153:errorcluster, "GenericScanMode out"=w143:refnum<class "ImagingModeDL090130Frame.lvclass">)  [unwired: 8 in]
            n144 = property on="settings" class="XSettings (strict)"(error in=w153, "Property"=TRUE ("is user-defined?")) -> (error out=w152:errorcluster)  [unwired: 1 in, 1 out]
            n145 = Scan From String(input string="update", error in=w152, default 1=internal_trigger_enum."update" ("internal trigger")) -> (error out=w150:errorcluster, output 1=w147:T4)  [unwired: 2 in, 2 out]
          }
          event "pixel dwell time": Value Change {
            n146 = event-data() -> ("CtlRef"=w176:refnum<vi>)  [unwired: 1 out]
            n147 = property class="DigNum (strict)"(reference=w176, error in=w175) -> (error out=w174:errorcluster, "Label.Text"=w173:string)  [unwired: 1 out]
            n148 = call "checkout.vi"("locked by?"=w173, "error in (no error)"=w174) -> ("GenericScanMode out"=w178:refnum<class "GenericImagingMode.lvclass">)  [unwired: 8 in, 1 out]
            n149 = To More Specific Class(target class=w172, reference=w178) -> (specific class reference=w181:refnum<class "ImagingModeDL090130Frame.lvclass">, error out=w182:errorcluster)  [unwired: 1 in]
            n150 = call-dynamic "set_speed_params.vi"("pixel-dwell time"="pixel dwell time", "error in (no error)"=w182, "ImagingModeDL090130Frame in"=w181) -> ("error out"=w179:errorcluster, "ImagingModeDL090130Frame out"=w180:refnum<class "ImagingModeDL090130Frame.lvclass">)  [unwired: 7 in]
            n151 = call-dynamic "checkin.vi"("error in (no error)"=w179, "GenericScanMode in"=w180) -> ("error out"=w165:errorcluster, "GenericScanMode out"=w177:refnum<class "ImagingModeDL090130Frame.lvclass">)  [unwired: 8 in]
            n152 = property on="settings" class="XSettings (strict)"(error in=w165, "Property"=TRUE ("is user-defined?")) -> (error out=w164:errorcluster)  [unwired: 1 in, 1 out]
            n153 = Scan From String(input string="update", error in=w164, default 1=internal_trigger_enum."update" ("internal trigger")) -> (error out=w169:errorcluster, output 1=w168:T4)  [unwired: 2 in, 2 out]
          }
          event "defineButton": Value Change {
            n154 = event-data() -> ("CtlRef"=w208:refnum<vi>)  [unwired: 1 out]
            n155 = property class="Bool"(reference=w208, error in=w209) -> (error out=w206:errorcluster, "Label.Text"=w207:string)  [unwired: 1 out]
            n156 = call "checkout.vi"("locked by?"=w207, "error in (no error)"=w206) -> ("error out"=w215:errorcluster, "GenericScanMode out"=w216:refnum<class "GenericImagingMode.lvclass">)  [unwired: 8 in]
            n157 = To More Specific Class(target class=w204, reference=w216, error in=w215) -> (specific class reference=w213:refnum<class "ImagingModeDL090130Frame.lvclass">, error out=w214:errorcluster)
            n158 = call-dynamic "get_Trajectory.vi"("error in (no error)"=w214, "ScanModeDL090923Scaffold in"=w213) -> ("error out"=w197:errorcluster, "Trajectory"=w198:refnum<class "GenericTrajectory.lvclass">, "ScanModeDL090923Scaffold out"=w210:refnum<class "ImagingModeDL090130Frame.lvclass">)  [unwired: 2 in, 5 out]
            n159 = call-dynamic "get_settings_cluster.vi"("error in (no error)"=w197, "GenericPlugin in"=w198) -> ("error out"=w196:errorcluster, "settings cluster"=w190:variant, "GenericPlugin out"=w195:refnum<class "GenericTrajectory.lvclass">)  [unwired: 7 in]
            n160 = call-dynamic "define.vi"("error in (no error)"=w196, "GenericTrajectory in"=w195) -> ("error out"=w191:errorcluster, "GenericTrajectory out"=w194:refnum<class "GenericTrajectory.lvclass">)  [unwired: 8 in]
            n161 = call-dynamic "get_settings_cluster.vi"("error in (no error)"=w191, "GenericPlugin in"=w194) -> ("error out"=w192:errorcluster, "settings cluster"=w189:variant, "GenericPlugin out"=w193:refnum<class "GenericTrajectory.lvclass">)  [unwired: 7 in]
            n162 = Not Equal?(x=w189, y=w190) -> (x != y?=w185:bool)
            n163 = call-dynamic "set_Trajectory.vi"("error in (no error)"=w192, "GenericTrajectory.lvclass"=w193, "ScanModeDL090923Scaffold in"=w210) -> ("error out"=w212:errorcluster, "ScanModeDL090923Scaffold out"=w211:refnum<class "ImagingModeDL090130Frame.lvclass">)  [unwired: 7 in]
            n164 = call-dynamic "checkin.vi"("error in (no error)"=w212, "GenericScanMode in"=w211) -> ("error out"=w188:errorcluster, "GenericScanMode out"=w205:refnum<class "ImagingModeDL090130Frame.lvclass">)  [unwired: 8 in]
            n165 = property on="settings" class="XSettings (strict)"(error in=w188) -> (error out=w187:errorcluster, "Property"=w186:bool)  [unwired: 1 in, 1 out]
            n166 = Or(x=w186, y=w185) -> (x .or. y?=w184:bool)
            n167 = property on="settings" class="XSettings (strict)"(error in=w187, "Property"=w184) -> (error out=w199:errorcluster)  [unwired: 1 in, 1 out]
            n168 = Scan From String(input string="update", error in=w199, default 1=internal_trigger_enum."update" ("internal trigger")) -> (error out=w201:errorcluster, output 1=w200:T4)  [unwired: 2 in, 2 out]
          }
          event "movie duration": Value Change {
            n169 = event-data() -> ()  [unwired: 2 out]
            n170 = call "obtain_latest_instance.vi"("error in (no error)"=w234) -> ("error out"=w233:errorcluster, "GenericScanMode out"=w231:refnum<class "GenericImagingMode.lvclass">)  [unwired: 9 in]
            n171 = To More Specific Class(target class=w226, reference=w231, error in=w233) -> (specific class reference=w230:refnum<class "ImagingModeDL090130Frame.lvclass">, error out=w232:errorcluster)
            n172 = call-dynamic "get_speed_params.vi"("error in (no error)"=w232, "ImagingModeDL090130Frame in"=w230) -> ("error out"=w221:errorcluster, "frame rate"=w229:dbl[unit], "ImagingModeDL090130Frame out"=w227:refnum<class "ImagingModeDL090130Frame.lvclass">)  [unwired: 4 in, 3 out]
            n173 = Multiply(x="movie duration", y=w229) -> (x*y=w225:dbl)
            n174 = local read "no. of averagings"() -> (w218:i32)
            n175 = To Double Precision Float(number=w218) -> (double precision float=w223:dbl)
            n176 = Divide(x=w225, y=w223) -> (x/y=w224:dbl)
            n177 = Round Toward +Infinity(x=w224) -> (ceil(x): smallest int >= x=w228:dbl)
            n178 = To Long Integer(number=w228) -> (32bit integer=w220:i32)
            n179 = property on="no. of frames" class="DigNum (strict)"(error in=w221, "Val(Sgnl)"=w220) -> (error out=w219:errorcluster)  [unwired: 1 in, 1 out]
          }
          event "x pixels", "y lines", "x aspect", "y aspect", "no. of frames", "no. of averagings", "step", "center\n (x galvo, V)", "amplitude\n (x galvo, V)", "center\n (y galvo, V)", "amplitude\n (y galvo, V)", "xy galvo view?": Value Change {
            n180 = event-data() -> ()  [unwired: 7 out]
            n181 = local write "enforce settings?"(FALSE ("settings enforced?")) -> ()
            n182 = call "checkout.vi"("locked by?"="parameter value change", "error in (no error)"=w257) -> ("error out"=w275:errorcluster, "GenericScanMode out"=w274:refnum<class "GenericImagingMode.lvclass">)  [unwired: 8 in]
            n183 = To More Specific Class(target class=w270, reference=w274, error in=w275) -> (specific class reference=w253:refnum<class "ImagingModeDL090130Frame.lvclass">, error out=w249:errorcluster)
            n184 = Unbundle By Name(w253) -> ("SpeedConstant"=w250:T3)
            n185 = case "What is kept constant?" shown="\"pixel dwell time\", Default" w250 {
              tunnel: [w278 w285 w290] -> w254
              tunnel: w253 -> [w280 w284 w288]
              tunnel: [w279 w283 w291] -> w252
              tunnel: w249 -> [w281 w286 w289]
              frame "pixel dwell time", Default {
                n186 = local read "pixel dwell time"() -> (w277:dbl[unit])
                n187 = call-dynamic "set_speed_params.vi"("pixel-dwell time"=w277, "error in (no error)"=w281, "ImagingModeDL090130Frame in"=w280) -> ("error out"=w278:errorcluster, "ImagingModeDL090130Frame out"=w279:refnum<class "ImagingModeDL090130Frame.lvclass">)  [unwired: 7 in]
              }
              frame "line scan time" {
                n188 = local read "line scan time"() -> (w282:dbl[unit])
                n189 = call-dynamic "set_speed_params.vi"("error in (no error)"=w286, "line-scan time"=w282, "ImagingModeDL090130Frame in"=w284) -> ("error out"=w285:errorcluster, "ImagingModeDL090130Frame out"=w283:refnum<class "ImagingModeDL090130Frame.lvclass">)  [unwired: 7 in]
              }
              frame "frame rate" {
                n190 = local read "frame rate"() -> (w287:dbl[unit])
                n191 = call-dynamic "set_speed_params.vi"("error in (no error)"=w289, "frame rate"=w287, "ImagingModeDL090130Frame in"=w288) -> ("error out"=w290:errorcluster, "ImagingModeDL090130Frame out"=w291:refnum<class "ImagingModeDL090130Frame.lvclass">)  [unwired: 7 in]
              }
            }
            n192 = Divide(x="amplitude\n (y galvo, V)", y=2.0) -> (x/y=w243:dbl)
            n193 = Add(x="center\n (y galvo, V)", y=w243) -> (x+y=→"Vmax(ygalvo)":dbl)
            n194 = Subtract(x="center\n (y galvo, V)", y=w243) -> (x-y=→"Vmin(ygalvo)":dbl)
            n195 = Divide(x="amplitude\n (x galvo, V)", y=2.0) -> (x/y=w247:dbl)
            n196 = Add(x="center\n (x galvo, V)", y=w247) -> (x+y=→"Vmax(xgalvo)":dbl)
            n197 = Subtract(x="center\n (x galvo, V)", y=w247) -> (x-y=→"Vmin(xgalvo)":dbl)
            n198 = Bundle By Name(cluster=w252, "xy galvo view?"="xy galvo view?", "ResolutionX"="x pixels", "ResolutionY"="y lines", "AspectRatioX"="x aspect", "AspectRatioY"="y aspect", "AveragingRepetitions"="no. of averagings", "Frames"="no. of frames", "StepSize"="step", "Vy0(V)"="center\n (x galvo, V)", "deltaVy(V)"="amplitude\n (x galvo, V)", "Vz0(V)"="center\n (y galvo, V)", "deltaVz(V)"="amplitude\n (y galvo, V)") -> (w251:refnum<class "ImagingModeDL090130Frame.lvclass">)
            n199 = property on="settings" class="XSettings (strict)"(error in=w254, "Property"=TRUE ("is user-defined?")) -> (error out=w255:errorcluster)  [unwired: 1 in, 1 out]
            n200 = call-dynamic "checkin.vi"("error in (no error)"=w255, "GenericScanMode in"=w251) -> ("error out"=w267:errorcluster, "GenericScanMode out"=w271:refnum<class "ImagingModeDL090130Frame.lvclass">)  [unwired: 8 in]
            n201 = Scan From String(input string="update", error in=w267, default 1=internal_trigger_enum."update" ("internal trigger")) -> (error out=w266:errorcluster, output 1=w265:T4)  [unwired: 2 in, 2 out]
          }
          event Value Change {
            n202 = event-data() -> ("CtlRef"=w303:refnum<vi>)  [unwired: 1 out]
            n203 = property class="Enum (strict)"(reference=w303, error in=w296) -> (error out=w295:errorcluster, "Label.Text"=w302:string)  [unwired: 1 out]
            n204 = call "checkout.vi"("locked by?"=w302, "error in (no error)"=w295) -> ("error out"=w305:errorcluster, "GenericScanMode out"=w304:refnum<class "GenericImagingMode.lvclass">)  [unwired: 8 in]
            n205 = To More Specific Class(target class=w301, reference=w304, error in=w305) -> (specific class reference=w299:refnum<class "ImagingModeDL090130Frame.lvclass">, error out=w300:errorcluster)
            n206 = Bundle By Name(cluster=w299, "SpeedConstant"="keep constant") -> (w297:refnum<class "ImagingModeDL090130Frame.lvclass">)
            n207 = call-dynamic "checkin.vi"("error in (no error)"=w300, "GenericScanMode in"=w297) -> ("error out"=w293:errorcluster)  [unwired: 8 in, 1 out]
            n208 = property on="settings" class="XSettings (strict)"(error in=w293, "Property"=TRUE ("is user-defined?")) -> (error out=w292:errorcluster)  [unwired: 1 in, 1 out]
          }
          event "enforce settings?": Value Change {
            n209 = event-data() -> ("CtlRef"=w318:refnum<vi>)  [unwired: 1 out]
            n210 = property class="Bool (strict)"(reference=w318, error in=w317) -> (error out=w316:errorcluster, "Label.Text"=w315:string)  [unwired: 1 out]
            n211 = call "checkout.vi"("locked by?"=w315, "error in (no error)"=w316) -> ("error out"=w341:errorcluster, "GenericScanMode out"=w340:refnum<class "GenericImagingMode.lvclass">)  [unwired: 8 in]
            n212 = To More Specific Class(target class=w339, reference=w340, error in=w341) -> (specific class reference=w321:refnum<class "ImagingModeDL090130Frame.lvclass">, error out=w323:errorcluster)
            n213 = local read "XIntensityCompensation"() -> (w312:cluster{"A":dbl, "lambda":dbl[unit], "C":dbl})
            n214 = local read "translation mode"() -> (w329:T2)
            n215 = local read "amplitude\n (y galvo, V)"() -> (w311:dbl)
            n216 = local read "amplitude\n (x galvo, V)"() -> (w309:dbl)
            n217 = local read "center\n (x galvo, V)"() -> (w308:dbl)
            n218 = local read "center\n (y galvo, V)"() -> (w310:dbl)
            n219 = local read "xy galvo view?"() -> (w307:bool)
            n220 = local read "no. of averagings"() -> (w332:i32)
            n221 = local read "return to origin?"() -> (w330:bool)
            n222 = local read "keep constant"() -> (w313:T3)
            n223 = local read "no. of frames"() -> (w333:i32)
            n224 = local read "x aspect"() -> (w335:dbl)
            n225 = local read "y aspect"() -> (w334:dbl)
            n226 = local read "x pixels"() -> (w337:i32)
            n227 = local read "y lines"() -> (w336:i32)
            n228 = local read "step"() -> (w331:dbl[unit])
            n229 = local read "frame rate"() -> (w319:dbl[unit])
            n230 = call-dynamic "set_speed_params.vi"("error in (no error)"=w323, "frame rate"=w319, "ImagingModeDL090130Frame in"=w321) -> ("error out"=w322:errorcluster, "ImagingModeDL090130Frame out"=w320:refnum<class "ImagingModeDL090130Frame.lvclass">)  [unwired: 7 in]
            n231 = Bundle By Name(cluster=w320, "ResolutionX"=w337, "ResolutionY"=w336, "AspectRatioX"=w335, "AspectRatioY"=w334, "SpeedConstant"=w313, "Frames"=w333, "AveragingRepetitions"=w332, "StepSize"=w331, "ReturnToOrigin"=w330, "TranslationMode"=w329, "IntensityCompensationParameters"=w312, "Vy0(V)"=w308, "deltaVy(V)"=w309, "Vz0(V)"=w310, "deltaVz(V)"=w311, "xy galvo view?"=w307) -> (w338:refnum<class "ImagingModeDL090130Frame.lvclass">)
            n232 = call-dynamic "checkin.vi"("error in (no error)"=w322, "GenericScanMode in"=w338) -> ("error out"=w326:errorcluster, "GenericScanMode out"=w314:refnum<class "ImagingModeDL090130Frame.lvclass">)  [unwired: 8 in]
            n233 = Scan From String(input string="update", error in=w326, default 1=internal_trigger_enum."update" ("internal trigger")) -> (error out=w325:errorcluster, output 1=w324:T4)  [unwired: 2 in, 2 out]
          }
          event Value Change {
            n234 = event-data() -> ("CtlRef"=w350:refnum<vi>)  [unwired: 1 out]
            n235 = property class="Enum (strict)"(reference=w350, error in=w349) -> (error out=w352:errorcluster, "Label.Text"=w351:string)  [unwired: 1 out]
            n236 = call "checkout.vi"("locked by?"=w351, "error in (no error)"=w352) -> ("error out"=w357:errorcluster, "GenericScanMode out"=w356:refnum<class "GenericImagingMode.lvclass">)  [unwired: 8 in]
            n237 = To More Specific Class(target class=w347, reference=w356, error in=w357) -> (specific class reference=w354:refnum<class "ImagingModeDL090130Frame.lvclass">, error out=w355:errorcluster)
            n238 = Bundle By Name(cluster=w354, "TranslationMode"="translation mode") -> (w353:refnum<class "ImagingModeDL090130Frame.lvclass">)
            n239 = call-dynamic "checkin.vi"("error in (no error)"=w355, "GenericScanMode in"=w353) -> ("error out"=w344:errorcluster, "GenericScanMode out"=w348:refnum<class "ImagingModeDL090130Frame.lvclass">)  [unwired: 8 in]
            n240 = property on="settings" class="XSettings (strict)"(error in=w344, "Property"=TRUE ("is user-defined?")) -> (error out=w343:errorcluster)  [unwired: 1 in, 1 out]
          }
          event Value Change {
            n241 = event-data() -> ()  [unwired: 2 out]
            n242 = Current VI's Path() -> (path=w361:path)
            n243 = call-dynamic "undock.vi"("error in (no error)"=w364, "undock?"="button:undock", "VI path"=w361, "component in"=w360) -> ("error out"=w363:errorcluster, "component out"=w359:refnum<class "ImagingModeDL090130Frame.lvclass">)  [unwired: 6 in]
          }
          event "XIntensityCompensation": Value Change {
            n244 = event-data() -> ("CtlRef"=w379:refnum<vi>)  [unwired: 1 out]
            n245 = property class="XIntensityCompensation (strict)"(reference=w379, error in=w372) -> (error out=w371:errorcluster, "Label.Text"=w376:string)  [unwired: 1 out]
            n246 = call "checkout.vi"("locked by?"=w376, "error in (no error)"=w371) -> ("error out"=w378:errorcluster, "GenericScanMode out"=w380:refnum<class "GenericImagingMode.lvclass">)  [unwired: 8 in]
            n247 = To More Specific Class(target class=w373, reference=w380, error in=w378) -> (specific class reference=w370:refnum<class "ImagingModeDL090130Frame.lvclass">, error out=w367:errorcluster)
            n248 = Bundle By Name(cluster=w370, "IntensityCompensationParameters"="XIntensityCompensation") -> (w375:refnum<class "ImagingModeDL090130Frame.lvclass">)
            n249 = property on="settings" class="XSettings (strict)"(error in=w367, "Property"=TRUE ("is user-defined?")) -> (error out=w366:errorcluster)  [unwired: 1 in, 1 out]
            n250 = call-dynamic "checkin.vi"("error in (no error)"=w366, "GenericScanMode in"=w375) -> ("error out"=w377:errorcluster, "GenericScanMode out"=w374:refnum<class "ImagingModeDL090130Frame.lvclass">)  [unwired: 8 in]
          }
          event "finished?": Value Change {
            n251 = event-data() -> ()  [unwired: 2 out]
          }
        }
        n252 = Unbundle By Name(w79) -> ("status"=w82:bool)
        n253 = To More Generic Class(target class=refnum<class "GenericComponent.lvclass"> refnum ("GenericComponent.lvclass"), reference=w70) -> (generic class reference=w73:refnum<class "GenericComponent.lvclass">)
        n254 = local write "settings"(w73) -> ()
        n255 = Or(x=w82, y=w81) -> (x .or. y?=w80:bool)
        n256 = To Variant(anything=w75) -> (Variant=w77:variant)
        n257 = call-dynamic "send_generic_trigger.vi"("error in (no error)"=w79, "trigger type"=trigger_type_enum."internal", "trigger variant"=w77, "GenericToplevelComponent in"=w70) -> ("error out"=w78:errorcluster, "GenericToplevelComponent out"=w71:refnum<class "ImagingModeDL090130Frame.lvclass">)  [unwired: 4 in, 2 out]
        "event error" <- w78
        "event handling loop counter" <- w83
      }
      n258 = call-dynamic "flush_trigger_queue.vi"("error in (no error)"=w41, "GenericToplevelComponent in"=w36) -> ("error out"=w40:errorcluster)  [unwired: 8 in, 1 out]
      n259 = property on="finished?" class="Bool (strict)"(error in=w61, "Val(Sgnl)"=w42) -> (error out=w56:errorcluster)  [unwired: 1 in, 1 out]
      n260 = call "send_error.vi"("additional message"="Error after event loop...", "error in (no error)"=w40) -> ("error out"=w50:errorcluster)  [unwired: 9 in]
      n261 = call "send_error.vi"("additional message"="Error after statemachine loop...", "error in (no error)"=w56) -> ("error out"=w54:errorcluster)  [unwired: 9 in]
      n262 = Merge Errors(w50, w54) -> (w52:errorcluster)
      n263 = call "checkout.vi"("locked by?"="", "error in (no error)"=w52) -> ("error out"=w51:errorcluster)  [unwired: 8 in, 1 out]
    }
    frame Error {
    }
  }
  "error out" <- w32
  "ImagingModeDL090130Frame out" <- w31
